vi "pid_motor.vi"(0 "kp":dbl, 1 "kd":dbl, 2 "ki":dbl, 3 "dt":dbl, 4 "err":dbl) -> (5 "u":dbl)   [LabVIEW 2019]
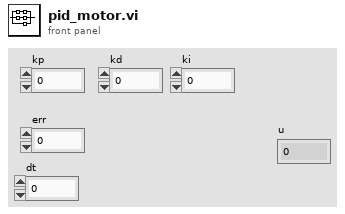
[diagram p1: front panel]
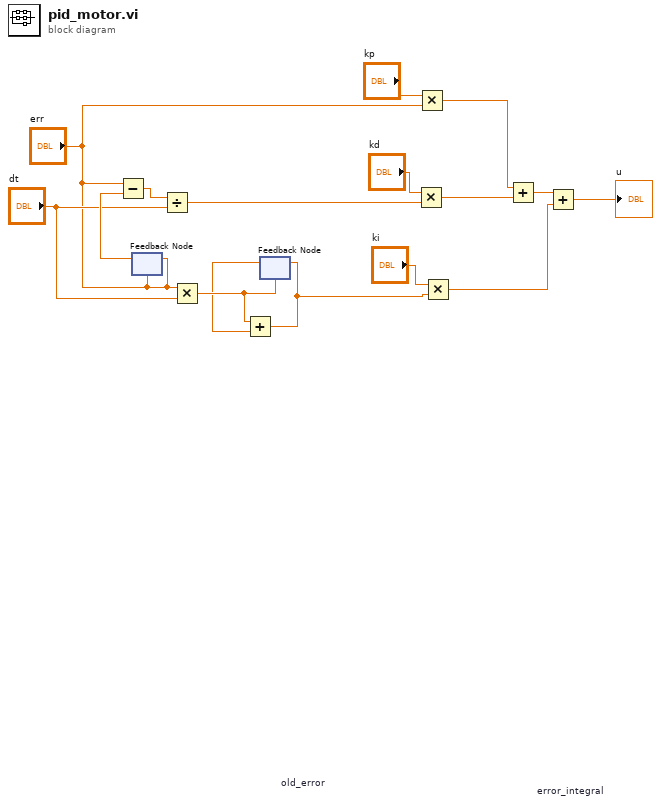
[diagram p0: block diagram]
diagram:
  n1 = feedback-in #1("err") -> ()
  n2 = feedback #1 "old_error"("err") -> (w16:dbl)
  n3 = Subtract(x="err", y=w16) -> (x-y=w15:dbl)
  n4 = Divide(x=w15, y="dt") -> (x/y=w8:dbl)
  n5 = Multiply(x="err", y="dt") -> (x*y=w13:dbl)
  n6 = feedback #2 "error_integral"(w13) -> (w12:dbl)
  n7 = Add(x=w13, y=w12) -> (x+y=w6:dbl)
  n8 = feedback-in #2(w6) -> ()
  n9 = Multiply(x="kd", y=w8) -> (x*y=w5:dbl)
  n10 = Multiply(x="kp", y="err") -> (x*y=w4:dbl)
  n11 = Multiply(x="ki", y=w6) -> (x*y=w2:dbl)
  n12 = Add(x=w4, y=w5) -> (x+y=w3:dbl)
  n13 = Add(x=w3, y=w2) -> (x+y=→"u":dbl)
